vi "Destroy.vi"(0 "Socket Communication in":refnum<class "Socket Communication.lvclass">, 5 "error in (no error)":errorcluster) -> (14 "Socket Communication out":refnum<class "Socket Communication.lvclass">, 19 "error out":errorcluster)   [LabVIEW 2016, in "Socket Communication.lvclass"]
uses:
  Socket Communication.lvclass
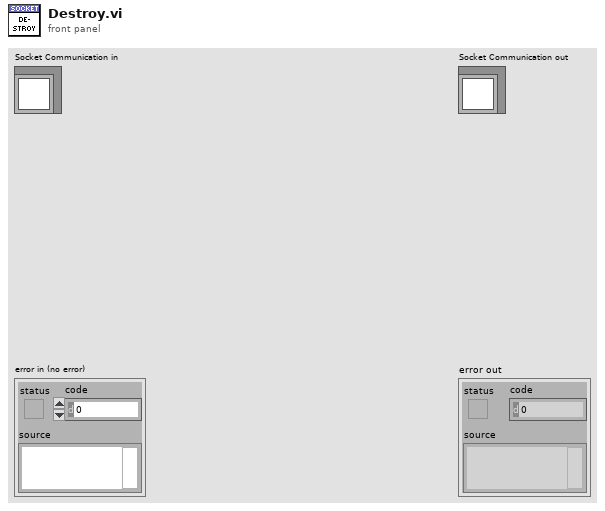
[diagram p1: front panel]
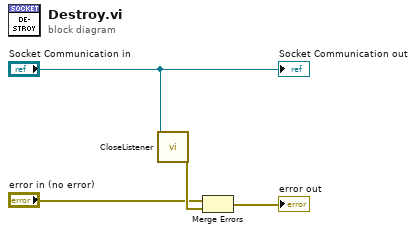
[diagram p0: block diagram]
diagram:
  n1 = call-dynamic "CloseListener.vi"("TCP Socket in"="Socket Communication in") -> ("error out"=w3:errorcluster)  [unwired: 17 in, 1 out]
  n2 = Merge Errors("error in (no error)", w3) -> (→"error out":errorcluster)
  "Socket Communication out" <- "Socket Communication in"
